vi "OnTaskCompleted.vi"(8 "error in (no error)":errorcluster, 10 "Correlation ID":u32, 11 "AutomationContext in":refnum<class "AutomationContext.lvclass">) -> (0 "error out":errorcluster, 3 "AutomationContext out":refnum<class "AutomationContext.lvclass">)   [LabVIEW 2023, in "Automation.lvlib" / "AutomationContext.lvclass"]
uses:
  AutomationContext.lvclass
  AutomationContext.lvclass/AutomationContext.ctl
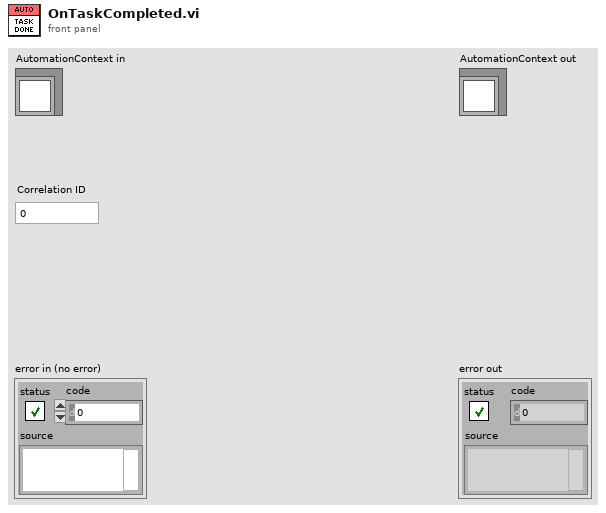
[diagram p1: front panel]
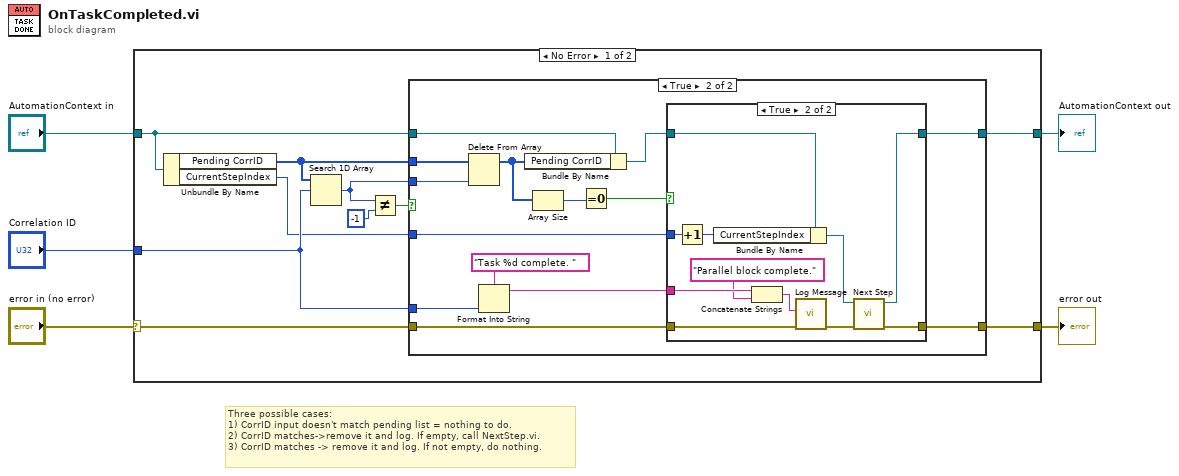
[diagram p0: block diagram]
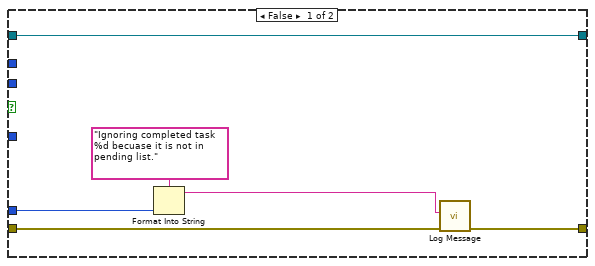
[diagram p2: hidden frame]
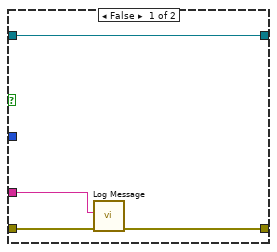
[diagram p3: hidden frame]
diagram:
  # "Three possible cases:\n1) CorrID input doesn't match pending list = nothing to do.\n2) CorrID matches->remove it and log. If empty, call NextStep.vi.\n3) CorrID matches -> remove it and log. If not empty, do nothing."
  n1 = case shown="No Error" "error in (no error)" {
    selector: "error in (no error)" -> [w15 w52]
    tunnel: [w14 w52] -> w4
    tunnel: [w13 w51] -> w2
    tunnel: "AutomationContext in" -> [w8 w51]
    tunnel: "Correlation ID" -> [w12 _]
    frame No Error {
      n2 = Unbundle By Name(w8) -> ("Pending CorrID"=w7:u32[], "CurrentStepIndex"=w9:u32)
      n3 = Search 1D Array(1D array=w7, element=w12) -> (index of element=w6:i32)  [unwired: 1 in]
      n4 = Not Equal?(x=w6, y=-1) -> (x != y?=w11:bool)
      n5 = case shown="True" w11 {
        tunnel: w15 -> [w19 w23]
        tunnel: [w20 w35] -> w14
        tunnel: [w21 w34] -> w13
        tunnel: w8 -> [w21 w33]
        tunnel: w12 -> [w16 w29]
        tunnel: w9 -> [_ w32]
        tunnel: w7 -> [_ w31]
        tunnel: w6 -> [_ w30]
        frame False {
          n6 = Format Into String(format string="Ignoring completed task %d becuase it is not in pending list.", w16) -> (resulting string=w18:string)  [unwired: 2 in, 1 out]
          n7 = call "Log Message.vi"("error constant"=w19, "input"=w18) -> ("error constant 2"=w20:errorcluster)  [unwired: 8 in, 1 out]
        }
        frame True {
          n8 = Delete From Array(array=w31, index=w30) -> (array with subset deleted=w26:u32[])  [unwired: 1 in, 1 out]
          n9 = Format Into String(format string="Task %d complete. ", w29) -> (resulting string=w22:string)  [unwired: 2 in, 1 out]
          n10 = Bundle By Name(cluster=w33, "Pending CorrID"=w26) -> (w27:refnum<class "AutomationContext.lvclass">)
          n11 = Array Size(array=w26) -> (size(s)=w25:i32)
          n12 = Equal To 0?(x=w25) -> (x = 0?=w24:bool)
          n13 = case shown="True" w24 {
            tunnel: [w37 w50] -> w35
            tunnel: [w39 w49] -> w34
            tunnel: w32 -> [_ w48]
            tunnel: w23 -> [w38 w44]
            tunnel: w27 -> [w39 w46]
            tunnel: w22 -> [w36 w42]
            frame False {
              n14 = call "Log Message.vi"("error constant"=w38, "input"=w36) -> ("error constant 2"=w37:errorcluster)  [unwired: 8 in, 1 out]
            }
            frame True {
              n15 = Increment(x=w48) -> (x+1=w47:u32)
              n16 = Bundle By Name(cluster=w46, "CurrentStepIndex"=w47) -> (w45:refnum<class "AutomationContext.lvclass">)
              n17 = Concatenate Strings(w42, "Parallel block complete." ("string")) -> (w41:string)
              n18 = call "Log Message.vi"("error constant"=w44, "input"=w41) -> ("error constant 2"=w43:errorcluster)  [unwired: 8 in, 1 out]
              n19 = call "Next Step.vi"("error in (no error)"=w43, "AutomationContext in"=w45) -> ("error out"=w50:errorcluster, "AutomationContext out"=w49:refnum<class "AutomationContext.lvclass">)  [unwired: 8 in]
            }
          }
        }
      }
    }
    frame Error {
    }
  }
  "error out" <- w4
  "AutomationContext out" <- w2
